vi "Coordinate_transforms.vi"(1 "Traverse Name":string="EnFlo Tunnel", 2 "Input":sgl[](array[numeric])=[0.0, 0.0, 0.0] format="%.2f", 3 "Mode":enum16{"XYZ to Channel", "Channel to XYZ"}(ring)) -> (0 "Output":sgl[](array[numeric]) format="%.2f")   [LabVIEW 2014]
uses:
  DriveConfigGlobal.vi
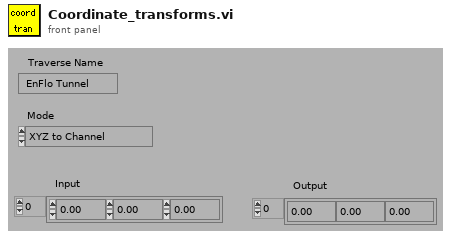
[diagram p1: front panel]
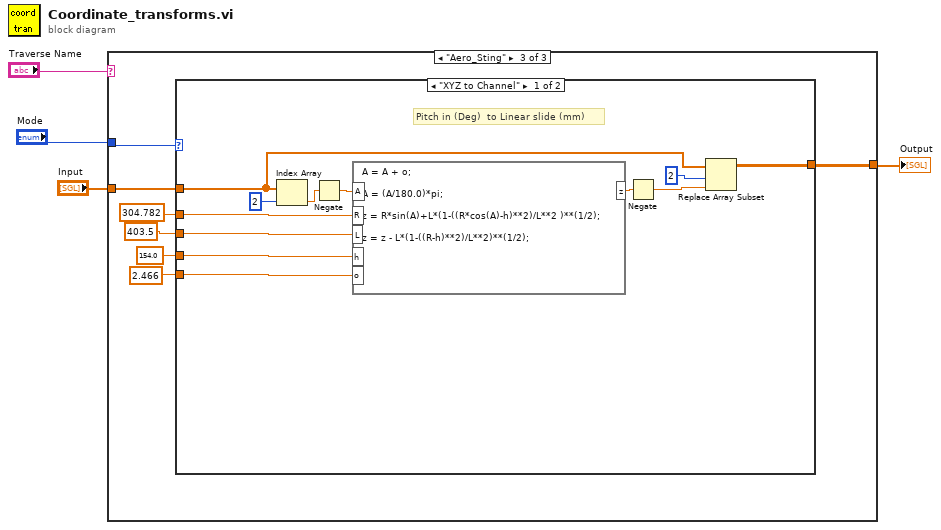
[diagram p0: block diagram]
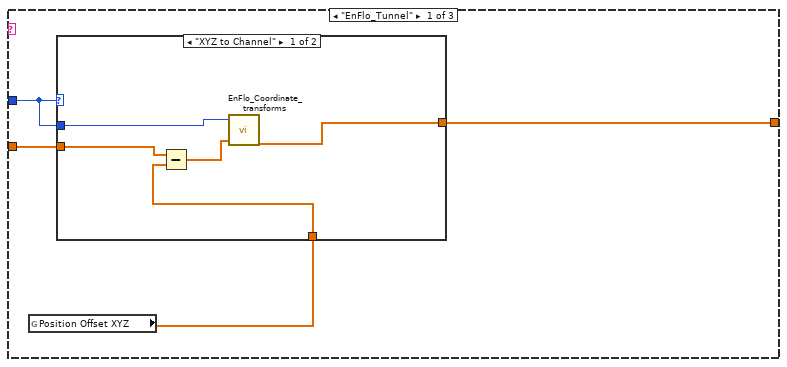
[diagram p2: hidden frame]
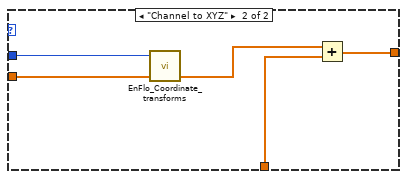
[diagram p3: hidden frame]
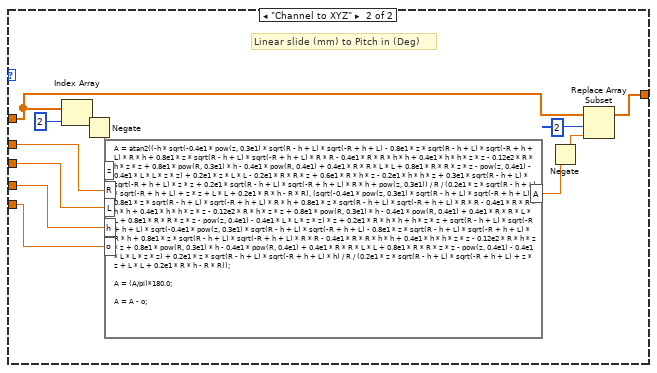
[diagram p5: hidden frame]
diagram:
  n1 = case shown="\"Aero_Sting\"" "Traverse Name" {
    tunnel: "Input" -> [w8 w19 w25]
    tunnel: [w6 w19 w24] -> w3
    tunnel: "Mode" -> [w5 _ w26]
    frame "EnFlo_Tunnel" {
      n2 = global read "DriveConfigGlobal.vi" "Position Offset XYZ"() -> (w7:dbl[])
      n3 = case shown="\"XYZ to Channel\"" w5 {
        tunnel: w8 -> [w11 w18]
        tunnel: w7 -> [w12 w16]
        tunnel: [w10 w15] -> w6
        tunnel: w5 -> [w9 w14]
        frame "XYZ to Channel" {
          n4 = Subtract(x=w11, y=w12) -> (x-y=w13:dbl[])
          n5 = call "EnFlo_Coordinate_transforms.vi"("Input"=w13, "Mode"=w9) -> ("Output"=w10:dbl[])  [unwired: 3 out]
        }
        frame "Channel to XYZ" {
          n6 = call "EnFlo_Coordinate_transforms.vi"("Input"=w18, "Mode"=w14) -> ("Output"=w17:dbl[])  [unwired: 3 out]
          n7 = Add(x=w17, y=w16) -> (x+y=w15:dbl[])
        }
      }
    }
    frame "D_Tunnel", Default {
    }
    frame "Aero_Sting" {
      n8 = case shown="\"XYZ to Channel\"" w26 {
        tunnel: w25 -> [w37 w42]
        tunnel: [w29 w41] -> w24
        tunnel: 2.466 -> [w35 w49]
        tunnel: 304.782 -> [w34 w50]
        tunnel: 403.5 -> [w33 w47]
        tunnel: 154.0 -> [w32 w48]
        frame "XYZ to Channel" {
          # "Pitch in (Deg)  to Linear slide (mm)"
          n9 = Index Array(array=w37, index=2) -> (element=w31:sgl)
          n10 = Negate(x=w31) -> (-x=w28:sgl)
          n11 = formula code="A = A + o;\n\nA = (A/180.0)*pi;\n\nz = R*sin(A)+L*(1-((R*cos(A)-h)**2)/L**2 )**(1/2);\n\nz = z - L*(1-((R-h)**2)/L**2)**(1/2);"("A"=w28, "R"=w34, "L"=w33, "h"=w32, "o"=w35) -> ("z"=w30:dbl)
          n12 = Negate(x=w30) -> (-x=w27:dbl)
          n13 = Replace Array Subset(array=w37, new element=w27, index=2) -> (w29:sgl[])
        }
        frame "Channel to XYZ" {
          # "Linear slide (mm) to Pitch in (Deg)"
          n14 = Index Array(array=w42, index=2) -> (element=w45:sgl)
          n15 = Negate(x=w45) -> (-x=w39:sgl)
          n16 = formula code="A = atan2((-h * sqrt(-0.4e1 * pow(z, 0.3e1) * sqrt(R - h + L) * sqrt(-R + h + L) - 0.8e1 * z * sqrt(R - h + L) * sqrt(-R + h + L) * R * h + 0.8e1 * z * sqrt(R - h + L) * sqrt(-R + h + L) * R * R - 0.4e1 * R * R * h * h + 0.4e1 * h * h * z * z - 0.12e2 * R * h * z * z + 0.8e1 * pow(R, 0.3e1) * h - 0.4e1 * pow(R, 0.4e1) + 0.4e1 * R * R * L * L + 0.8e1 * R * R * z * z - pow(z, 0.4e1) - 0.4e1 * L * L * z * z) + 0.2e1 * z * L * L - 0.2e1 * R * R * z + 0.6e1 * R * h * z - 0.2e1 * h * h * z + 0.3e1 * sqrt(R - h + L) * sqrt(-R + h + L) * z * z + 0.2e1 * sqrt(R - h + L) * sqrt(-R + h + L) * R * h + pow(z, 0.3e1)) / R / (0.2e1 * z * sqrt(R - h + L) * sqrt(-R + h + L) + z * z + L * L + 0.2e1 * R * h - R * R), (sqrt(-0.4e1 * pow(z, 0.3e1) * sqrt(R - h + L) * sqrt(-R + h + L) - 0.8e1 * z * sqrt(R - h + L) * sqrt(-R + h + L) * R * h + 0.8e1 * z * sqrt(R - h + L) * sqrt(-R + h + L) * R * R - 0.4e1 * R * R * h * h + 0.4e1 * h * h * z * z - 0.12e2 * R * h * z * z + 0.8e1 * pow(R, 0.3e1) * h - 0.4e1 * pow(R, 0.4e1) + 0.4e1 * R * R * L * L + 0.8e1 * R * R * z * z - pow(z, 0.4e1) - 0.4e1 * L * L * z * z) * z + 0.2e1 * R * h * h + h * z * z + sqrt(R - h + L) * sqrt(-R + h + L) * sqrt(-0.4e1 * pow(z, 0.3e1) * sqrt(R - h + L) * sqrt(-R + h + L) - 0.8e1 * z * sqrt(R - h + L) * sqrt(-R + h + L) * R * h + 0.8e1 * z * sqrt(R - h + L) * sqrt(-R + h + L) * R * R - 0.4e1 * R * R * h * h + 0.4e1 * h * h * z * z - 0.12e2 * R * h * z * z + 0.8e1 * pow(R, 0.3e1) * h - 0.4e1 * pow(R, 0.4e1) + 0.4e1 * R * R * L * L + 0.8e1 * R * R * z * z - pow(z, 0.4e1) - 0.4e1 * L * L * z * z) + 0.2e1 * z * sqrt(R - h + L) * sqrt(-R + h + L) * h) / R / (0.2e1 * z * sqrt(R - h + L) * sqrt(-R + h + L) + z * z + L * L + 0.2e1 * R * h - R * R));\n\nA = (A/pi)*180.0;\n\nA = A - o;"("z"=w39, "R"=w50, "L"=w47, "h"=w48, "o"=w49) -> ("A"=w43:dbl)
          n17 = Negate(x=w43) -> (-x=w40:dbl)
          n18 = Replace Array Subset(array=w42, new element=w40, index=2) -> (w41:sgl[])
        }
      }
    }
  }
  "Output" <- w3
